vi "Find Range Check Result.vi"   [LabVIEW 2013, in "ACNET Monitor.lvlib"]
uses:
  ACNET Monitor.lvlib
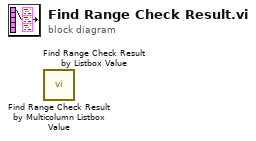
[diagram p0: block diagram]
diagram:
  n1 = call "Find Range Check Result by Multicolumn Listbox Value.vi"() -> ()  [unwired: 3 in, 3 out]
  n2 = call "Find Range Check Result by Listbox Value.vi"() -> ()  [unwired: 3 in, 3 out]
